vi "Main.vi"() -> ()   [LabVIEW 2021]
doc: "Use this template to build a simple state machine design pattern. Each state executes code and determines which state to transition to."
uses:
  controls/State.ctl
  controls/Data.ctl
  vmmso/vmmso.lvlib
panel:
  in  "Amplitude":dbl
  in  "Bias":dbl
  in  "Freq":dbl
  in  "Wave Style":u16(ring) items=["Sine", "Square", "Ramp"]
  out "Is Data Ready？":bool
  out "ReadVoltageData Return":u32
  out "Voltage Wave":dbl[](graph)
  out "Capture Return":i32
  out "Device is OK?":bool
  out "Support Samples":u32[](array[numeric])
  in  "Exit":bool
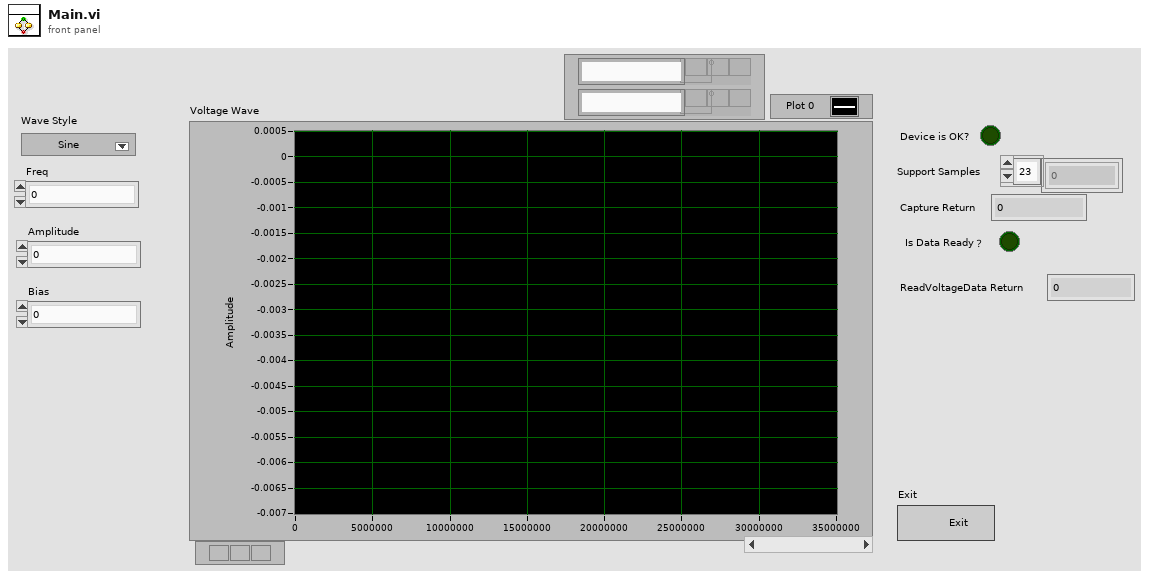
[diagram p1: front panel]
types:
  T1 = typedef "Data.ctl" = cluster{"Boolean <Replace Me>":bool, "String <Replace Me>":string, "Numeric <Replace Me>":dbl}
  T2 = typedef "State.ctl" = enum16{"Initialize", "Wait for UsbIn", "Init Osc and Dds", "Wait for Event", "Capture", "Read Voltage", "Exit"}
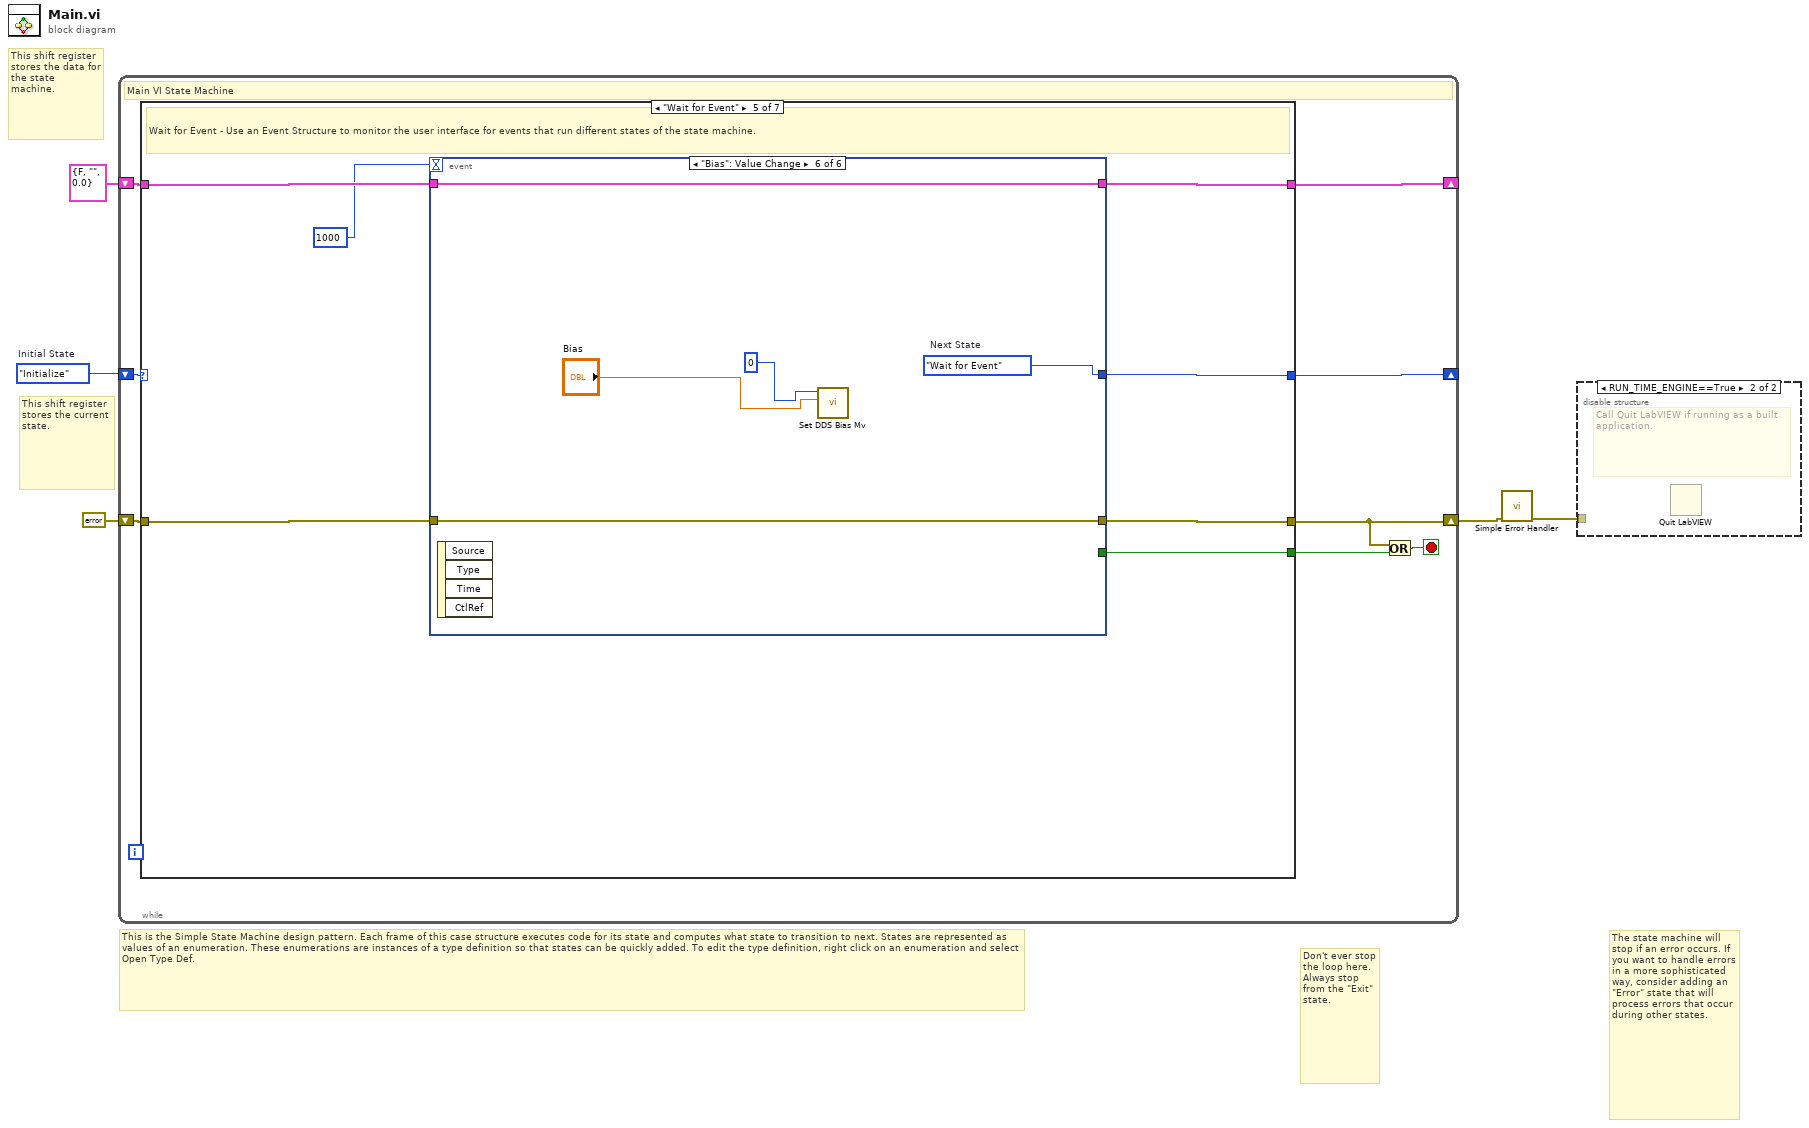
[diagram p0: block diagram]
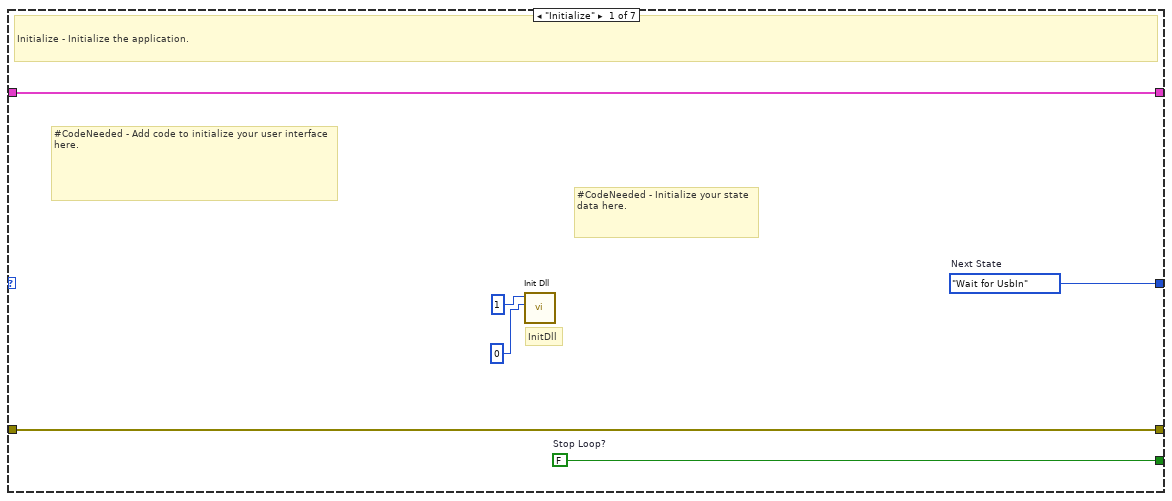
[diagram p3: hidden frame]
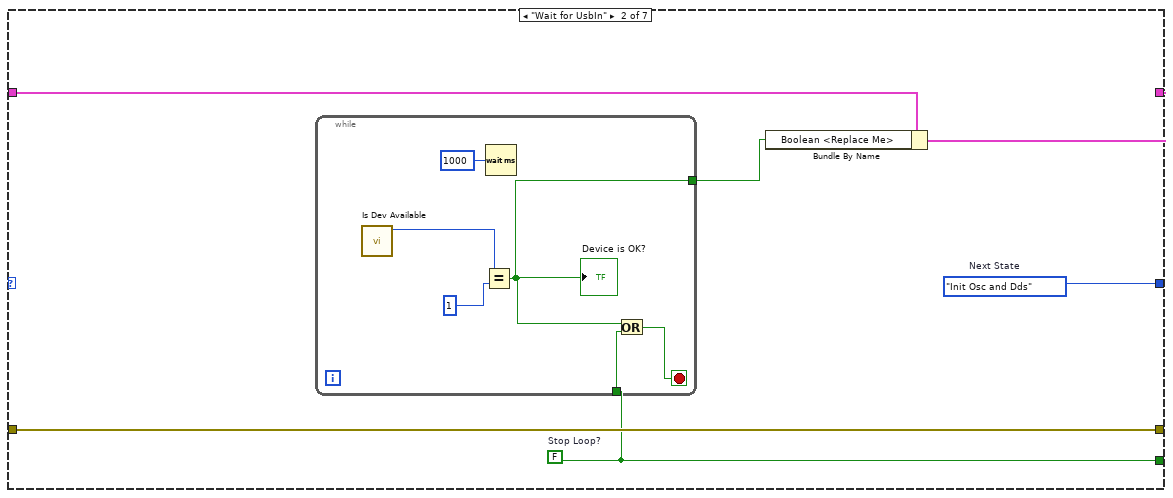
[diagram p4: hidden frame]
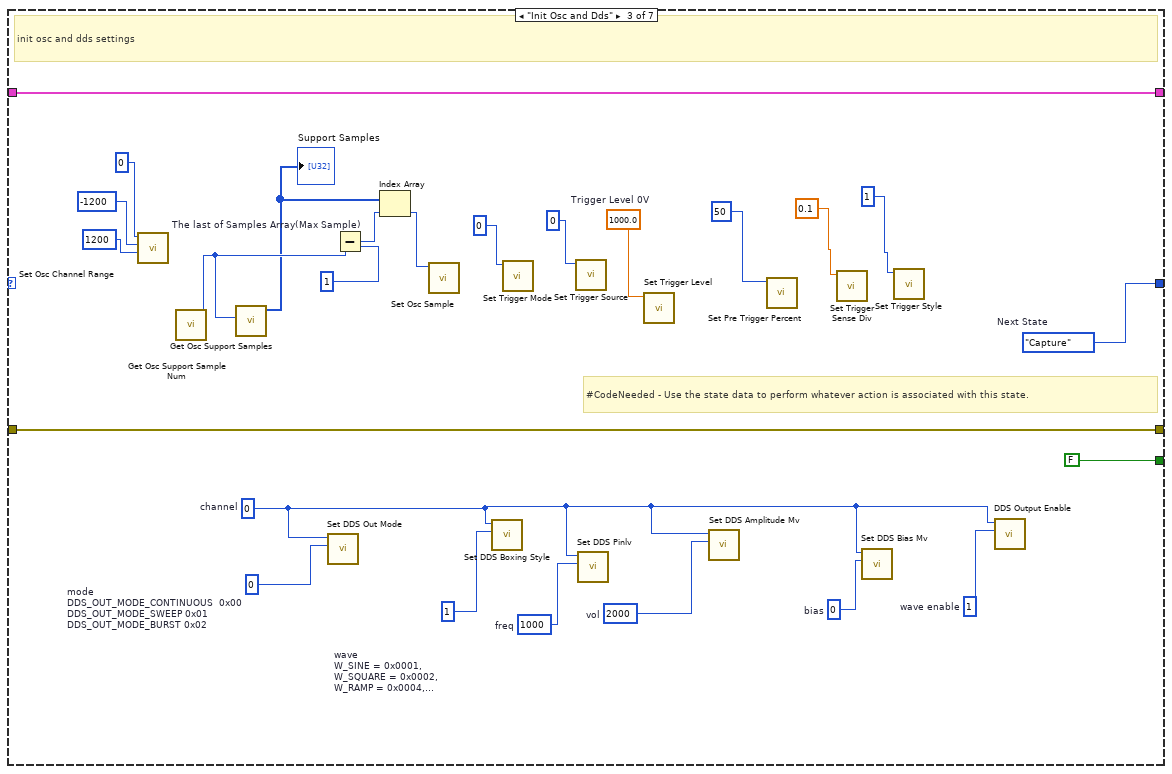
[diagram p5: hidden frame]
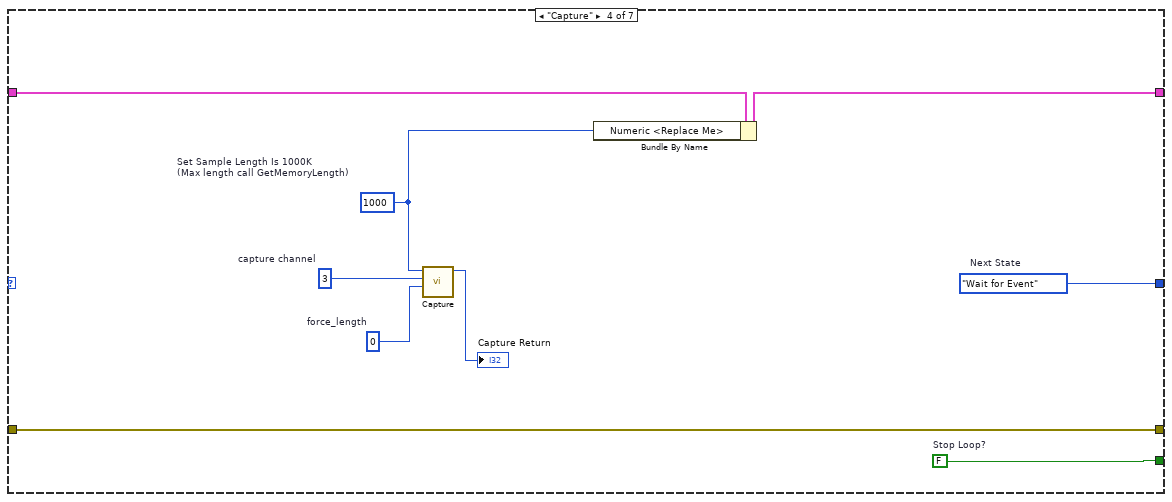
[diagram p6: hidden frame]
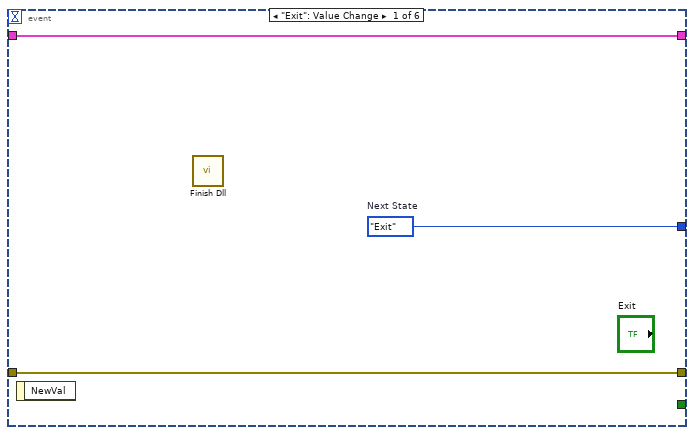
[diagram p7: hidden frame]
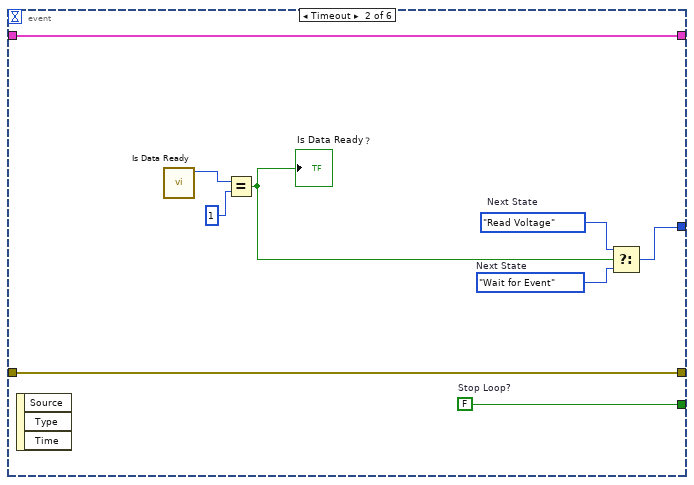
[diagram p8: hidden frame]
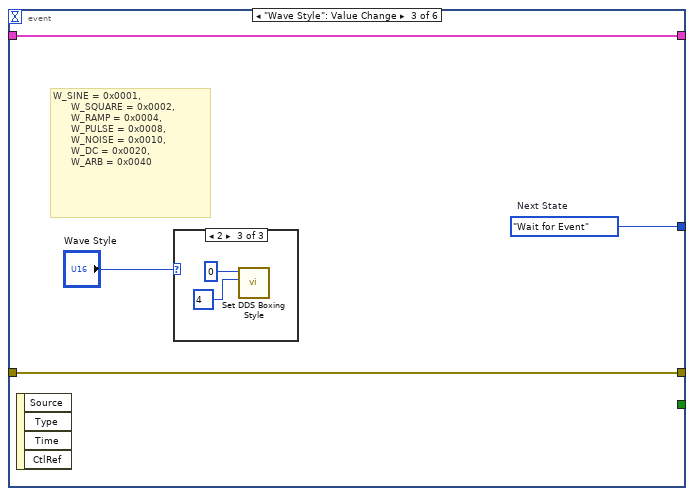
[diagram p9: hidden frame]
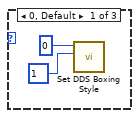
[diagram p10: hidden frame]
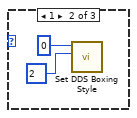
[diagram p11: hidden frame]
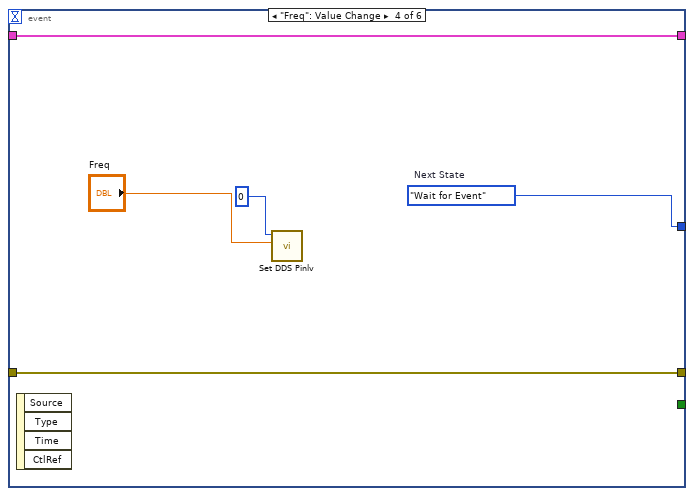
[diagram p12: hidden frame]
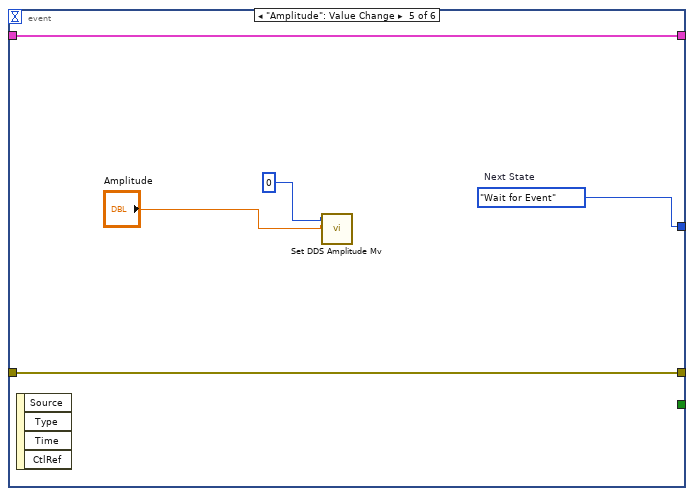
[diagram p13: hidden frame]
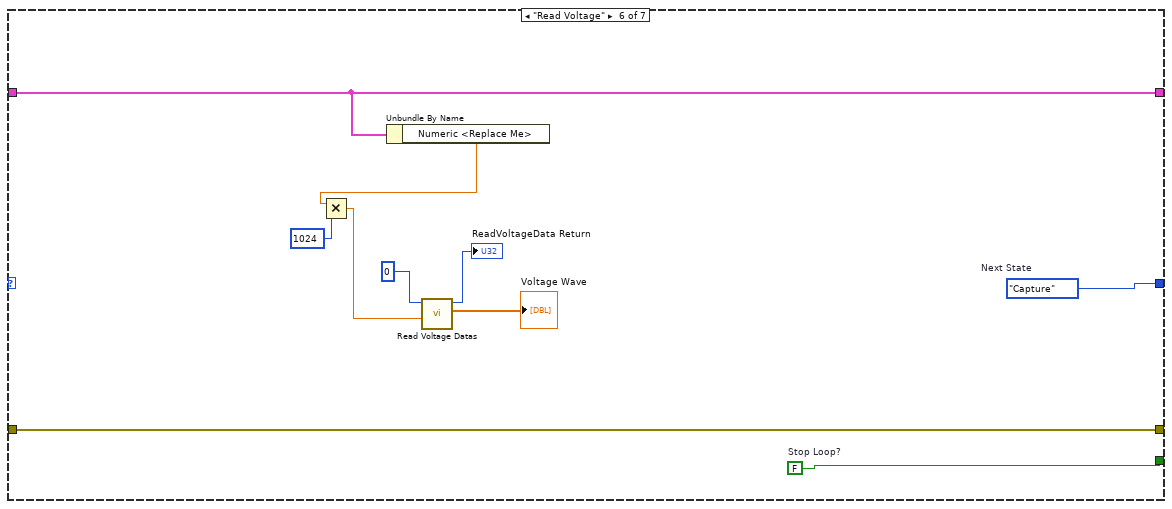
[diagram p14: hidden frame]
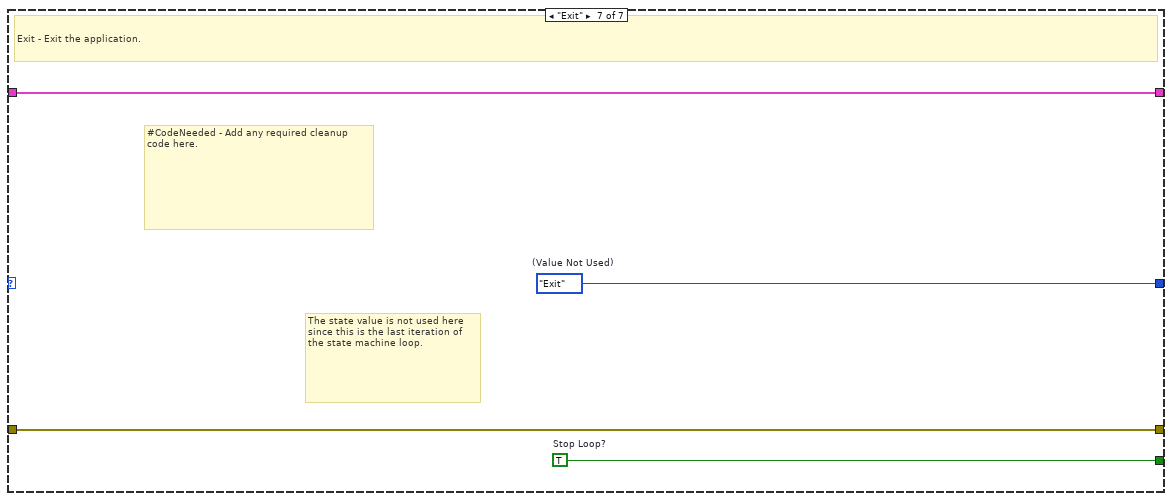
[diagram p15: hidden frame]
diagram:
  w5 = State."Initialize"  # Initial State
  # "Don't ever stop the loop here. Always stop from the \"Exit\" state."
  # "The state machine will stop if an error occurs. If you want to handle errors in a more sophisticated way, consider adding an \"Error\" state that will process errors that occur during other states."
  # "This shift register stores the data for the state machine."
  # "This is the Simple State Machine design pattern. Each frame of this case structure executes code for its state and computes what state to transition to next. States are represented as values of an enumeration. These enumerations are instances of a type definition so that states can be quickly added. To edit the type definition, right click on an enumeration and select Open Type Def."
  # "This shift register stores the current state."
  n1 = while {
    shift-right: [w12] -> _
    shift-left: w5 -> [w13]
    shift-right: [w10] -> _
    shift-left: T1 {"Boolean <Replace Me>"=FALSE, "String <Replace Me>"="", "Numeric <Replace Me>"=0.0} ("Data") -> [w11]
    shift-right: [w7] -> w2
    shift-left: errorcluster {"status"=FALSE, "code"=0, "source"=""} ("error constant") -> [w9]
    stop <- w8 stop-if-true
    # "Main VI State Machine"
    n2 = case shown="\"Wait for Event\"" w13 {
      tunnel: [w19 w24 w56 w64 w72 w117 w123] -> w12
      tunnel: w11 -> [w14 w22 w54 w59 w71 w111 w122]
      tunnel: [w14 w21 w54 w58 w70 w111 w122] -> w10
      tunnel: w9 -> [w17 w25 w53 w65 w69 w119 w120]
      tunnel: [w17 w25 w53 w65 w68 w119 w120] -> w7
      tunnel: [w18 w23 FALSE ("Stop Loop?") w63 w67 w118 w121] -> w6
      frame "Initialize" {
        w18 = FALSE  # Stop Loop?
        w19 = State."Wait for UsbIn"  # Next State
        # "InitDll"
        # "#CodeNeeded - Initialize your state data here."
        # "#CodeNeeded - Add code to initialize your user interface here."
        # "Initialize - Initialize the application."
        n3 = call "Init Dll.vi"("en_hard_watchdog"=0 ("channel"), "en_log"=1 ("channel")) -> ()  [unwired: 9 in, 1 out]
      }
      frame "Wait for UsbIn" {
        w24 = State."Init Osc and Dds"  # Next State
        w23 = FALSE  # Stop Loop?
        n4 = while {
          tunnel: w23 -> [w29]
          tunnel: [w26] -> w20
          stop <- w28 stop-if-true
          n5 = call "Is Dev Available.vi"() -> ("function return"=w27:i32)  [unwired: 11 in]
          n6 = Equal?(x=w27, y=1 ("channel")) -> (x = y?=w26:bool)
          "Device is OK?" <- w26
          n7 = Wait (ms)(milliseconds to wait=u32 1000 ("等待时间（毫秒）")) -> ()  [unwired: 1 out]
          n8 = Or(x=w26, y=w29) -> (x .or. y?=w28:bool)
        }
        n9 = Bundle By Name(cluster=w22, "Boolean <Replace Me>"=w20) -> (w21:T1)
      }
      frame "Init Osc and Dds" {
        w32 = i8 0  # mode DDS_OUT_MODE_CONTINUOUS  0x00 DDS_OUT_MODE_SWEEP 0x01 DDS_OUT_MODE_BURST 0x02
        w34 = i8 1  # wave enable
        w36 = u32 0  # bias
        w35 = u32 2000  # vol
        w37 = u32 1000  # freq
        w38 = i8 1  # wave  W_SINE = 0x0001,  W_SQUARE = 0x0002,  W_RAMP = 0x0004,  W_PULSE = 0x0008,  W_NOISE = 0x0010,  W_DC = 0x0020,  W_ARB = 0x0040
        w33 = i8 0  # channel
        w48 = sgl 1000.0  # Trigger Level 0V
        w56 = State."Capture"  # Next State
        # "#CodeNeeded - Use the state data to perform whatever action is associated with this state."
        # "init osc and dds settings"
        n10 = call "Set Osc Channel Range.vi"("maxmv"=1200 ("minmv"), "minmv"=-1200, "channel"=0) -> ()  [unwired: 8 in, 1 out]
        n11 = call "Get Osc Support Sample Num.vi"() -> ("function return"=w44:i32)  [unwired: 11 in]
        n12 = call "Get Osc Support Samples.vi"("maxnum"=w44) -> ("sample out"=w41:u32[])  [unwired: 9 in, 1 out]
        "Support Samples" <- w41
        n13 = call "Set DDS Out Mode.vi"("out_mode"=w32, "channel_index"=w33) -> ()  [unwired: 10 in]
        n14 = Subtract "The last of Samples Array(Max Sample)"(x=w44, y=1 ("front")) -> (x-y=w46:i32)
        n15 = Index Array(array=w41, index=w46) -> (element=w47:u32)
        n16 = call "Set Osc Sample.vi"("sample"=w47) -> ()  [unwired: 10 in, 1 out]
        n17 = call "Set DDS Boxing Style.vi"("boxing"=w38, "channel_index"=w33) -> ()  [unwired: 10 in]
        n18 = call "Set Trigger Mode.vi"("mode"=0 ("front")) -> ()  [unwired: 11 in]
        n19 = call "Set Trigger Source.vi"("source"=0 ("front")) -> ()  [unwired: 11 in]
        n20 = call "Set DDS Pinlv.vi"("pinlv"=w37, "channel_index"=w33) -> ()  [unwired: 10 in]
        n21 = call "Set Trigger Level.vi"("level"=w48) -> ()  [unwired: 11 in]
        n22 = call "Set DDS Amplitude Mv.vi"("amplitdude"=w35, "channel_index"=w33) -> ()  [unwired: 10 in]
        n23 = call "Set Pre Trigger Percent.vi"("front"=50) -> ()  [unwired: 11 in]
        n24 = call "Set Trigger Sense Div.vi"("sense"=0.1) -> ()  [unwired: 11 in]
        n25 = call "Set DDS Bias Mv.vi"("bias"=w36, "channel_index"=w33) -> ()  [unwired: 10 in]
        n26 = call "Set Trigger Style.vi"("style"=u32 1) -> ()  [unwired: 11 in]
        n27 = call "DDS Output Enable.vi"("enable"=w34, "channel_index"=w33) -> ()  [unwired: 10 in]
      }
      frame "Capture" {
        w60 = i8 0  # force_length
        w57 = u32 1000  # Set Sample Length Is 1000K (Max length call GetMemoryLength)
        w61 = i8 3  # capture channel
        w63 = FALSE  # Stop Loop?
        w64 = State."Wait for Event"  # Next State
        n28 = call "Capture.vi"("force_length"=w60, "capture_channel"=w61, "length"=w57) -> ("function return"=→"Capture Return":i32)  [unwired: 8 in]
        n29 = Bundle By Name(cluster=w59, "Numeric <Replace Me>"=w57) -> (w58:T1)
      }
      frame "Wait for Event" {
        # "Wait for Event - Use an Event Structure to monitor the user interface for events that run different states of the state machine."
        n30 = event shown="[5] \"Bias\": Value Change" {
          selector: _ -> [_ _ _ _ _ _]
          dyn-events: _ -> [_ _ _ _ _ _]
          timeout: 1000 ("y") -> [_ _ _ _ _ _]
          tunnel: [w75 w79 w85 w97 w102 w107] -> w72
          tunnel: w71 -> [w74 w84 w88 w99 w104 w109]
          tunnel: [w74 w84 w88 w99 w104 w109] -> w70
          tunnel: w69 -> [w73 w83 w87 w98 w103 w108]
          tunnel: [w73 w83 w87 w98 w103 w108] -> w68
          tunnel: [_ w80 _ _ _ _] -> w67
          event "Exit": Value Change {
            w75 = State."Exit"  # Next State
            n31 = event-data() -> ()  [unwired: 1 in, 1 out]
            n32 = call "Finish Dll.vi"() -> ()  [unwired: 11 in, 1 out]
          }
          event Timeout {
            w76 = State."Wait for Event"  # Next State
            w80 = FALSE  # Stop Loop?
            w77 = State."Read Voltage"  # Next State
            n33 = event-data() -> ()  [unwired: 1 in, 3 out]
            n34 = call "Is Data Ready.vi"() -> ("function return"=w82:i32)  [unwired: 11 in]
            n35 = Equal?(x=w82, y=1) -> (x = y?=w78:bool)
            "Is Data Ready？" <- w78
            n36 = Select(t=w77, s=w78, f=w76) -> (s? t:f=w79:T2)
          }
          event "Wave Style": Value Change {
            w85 = State."Wait for Event"  # Next State
            # "W_SINE = 0x0001, \n\t\t\t\t\t\tW_SQUARE = 0x0002, \n\t\t\t\t\t\tW_RAMP = 0x0004, \n\t\t\t\t\t\tW_PULSE = 0x0008, \n\t\t\t\t\t\tW_NOISE = 0x0010, \n\t\t\t\t\t\tW_DC = 0x0020, \n\t\t\t\t\t\tW_ARB = 0x0040"
            n37 = event-data() -> ()  [unwired: 1 in, 4 out]
            n38 = case shown="2" "Wave Style" {
              frame 0, Default {
                n39 = call "Set DDS Boxing Style.vi"("boxing"=1 ("y"), "channel_index"=0 ("y")) -> ()  [unwired: 10 in]
              }
              frame 1 {
                n40 = call "Set DDS Boxing Style.vi"("boxing"=2 ("y"), "channel_index"=0 ("y")) -> ()  [unwired: 10 in]
              }
              frame 2 {
                n41 = call "Set DDS Boxing Style.vi"("boxing"=4 ("y"), "channel_index"=0 ("y")) -> ()  [unwired: 10 in]
              }
            }
          }
          event "Freq": Value Change {
            w97 = State."Wait for Event"  # Next State
            n42 = event-data() -> ()  [unwired: 1 in, 4 out]
            n43 = call "Set DDS Pinlv.vi"("pinlv"="Freq", "channel_index"=0 ("y")) -> ()  [unwired: 10 in]
          }
          event "Amplitude": Value Change {
            w102 = State."Wait for Event"  # Next State
            n44 = event-data() -> ()  [unwired: 1 in, 4 out]
            n45 = call "Set DDS Amplitude Mv.vi"("amplitdude"="Amplitude", "channel_index"=0 ("y")) -> ()  [unwired: 10 in]
          }
          event "Bias": Value Change {
            w107 = State."Wait for Event"  # Next State
            n46 = event-data() -> ()  [unwired: 1 in, 4 out]
            n47 = call "Set DDS Bias Mv.vi"("bias"="Bias", "channel_index"=0 ("y")) -> ()  [unwired: 10 in]
          }
        }
      }
      frame "Read Voltage" {
        w117 = State."Capture"  # Next State
        w118 = FALSE  # Stop Loop?
        n48 = Unbundle By Name(w111) -> ("Numeric <Replace Me>"=w110:dbl)
        n49 = Multiply(x=w110, y=1024) -> (x*y=w113:dbl)
        n50 = call "Read Voltage Datas.vi"("length"=w113, "channel"=i8 0) -> ("buffer out"=→"Voltage Wave":dbl[], "function return"=→"ReadVoltageData Return":u32)  [unwired: 8 in]
      }
      frame "Exit" {
        w121 = TRUE  # Stop Loop?
        w123 = State."Exit"  # (Value Not Used)
        # "#CodeNeeded - Add any required cleanup code here."
        # "The state value is not used here since this is the last iteration of the state machine loop."
        # "Exit - Exit the application."
      }
    }
    n51 = Or(x=w7, y=w6) -> (x .or. y?=w8:bool)
  }
  n52 = call <vilib>:"Simple Error Handler.vi"("error in (no error)"=w2) -> ("error out"=w1:errorcluster)  [unwired: 4 in, 4 out]
  n53 = disable-structure shown="RUN_TIME_ENGINE==True" {
    disable-tunnel: w1 -> [_ _]
    frame condition #0 (active) {
    }
    frame condition #1 {
      # "Call Quit LabVIEW if running as a built application."
      n54 = Quit LabVIEW() -> ()  [unwired: 1 in]
    }
  }
